vi "3d axis settings.vi"(3 "Int Current":T1, 4 "Wave Current":T1, 5 "Scan Current":T1) -> (0 "Int setting":T1, 1 "Wave setting":T1, 2 "Scan setting":T1)   [LabVIEW 2014]
panel:
  in  "Save":bool
  in  "Cancel":bool
  in  "Int Auto":bool caption="Auto"
  in  "Int Min":sgl caption="Min"
  in  "Int Max":sgl caption="Max"
  in  "Wave Auto":bool caption="Auto"
  in  "Wave Min":sgl caption="Min"
  in  "Wave Max":sgl caption="Max"
  in  "Scan Auto":bool caption="Auto"
  in  "Scan Min":sgl caption="Min"
  in  "Scan Max":sgl caption="Max"
  # "Int plot Axis scale"
  # "Wavelength"
  # "Scan"
  # "Intensity"
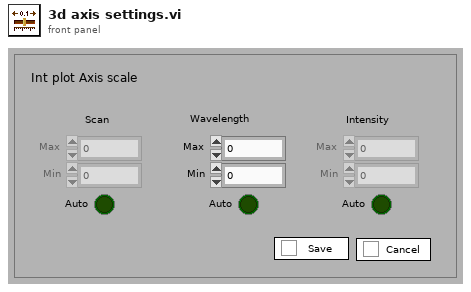
[diagram p1: front panel]
types:
  T1 = cluster{"ZScale.Maximum":dbl, "ZScale.Minimum":dbl, "ZScale.ScaleFit":u8}
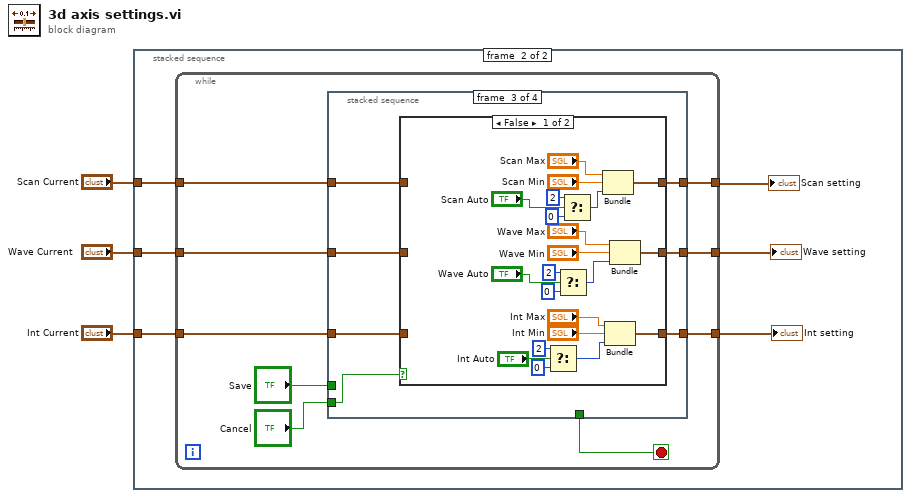
[diagram p0: block diagram]
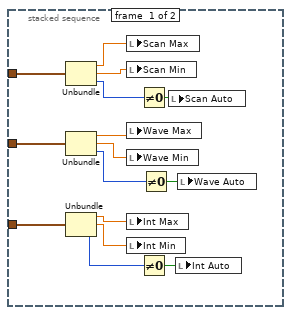
[diagram p2: hidden frame]
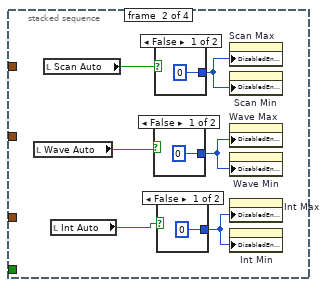
[diagram p4: hidden frame]
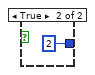
[diagram p5: hidden frame]
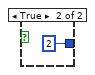
[diagram p6: hidden frame]
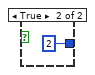
[diagram p7: hidden frame]
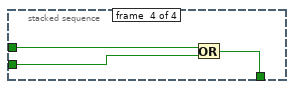
[diagram p9: hidden frame]
diagram:
  n1 = stacked-sequence {
    tunnel: "Scan Current" -> [w18 w24]
    tunnel: "Wave Current" -> [w17 w23]
    tunnel: "Int Current" -> [w16 w22]
    frame #0 {
      n2 = Unbundle(w18) -> ("ZScale.Maximum"=w15:dbl, "ZScale.Minimum"=w14:dbl, "ZScale.ScaleFit"=w9:u8)
      n3 = Unbundle(w17) -> ("ZScale.Maximum"=w13:dbl, "ZScale.Minimum"=w12:dbl, "ZScale.ScaleFit"=w7:u8)
      n4 = Unbundle(w16) -> ("ZScale.Maximum"=w11:dbl, "ZScale.Minimum"=w10:dbl, "ZScale.ScaleFit"=w5:u8)
      n5 = local write "Scan Max"(w15) -> ()
      n6 = local write "Scan Min"(w14) -> ()
      n7 = local write "Wave Max"(w13) -> ()
      n8 = local write "Wave Min"(w12) -> ()
      n9 = local write "Int Max"(w11) -> ()
      n10 = local write "Int Min"(w10) -> ()
      n11 = Not Equal To 0?(x=w9) -> (x != 0?=w8:bool)
      n12 = Not Equal To 0?(x=w5) -> (x != 0?=w4:bool)
      n13 = Not Equal To 0?(x=w7) -> (x != 0?=w6:bool)
      n14 = local write "Scan Auto"(w8) -> ()
      n15 = local write "Int Auto"(w4) -> ()
      n16 = local write "Wave Auto"(w6) -> ()
    }
    frame #1 {
      n17 = while {
        tunnel: [w33] -> w21
        tunnel: [w29] -> w20
        tunnel: [w28] -> w19
        tunnel: w24 -> [w27]
        tunnel: w23 -> [w26]
        tunnel: w22 -> [w25]
        stop <- w32 stop-if-true
        n18 = stacked-sequence {
          tunnel: [_ _ w52 _] -> w33
          tunnel: [_ _ _ w79] -> w32
          tunnel: "Cancel" -> [_ _ w49 w78]
          tunnel: "Save" -> [_ _ _ w77]
          tunnel: [_ _ w51 _] -> w29
          tunnel: [_ _ w50 _] -> w28
          tunnel: w27 -> [_ _ w48 _]
          tunnel: w26 -> [_ _ w47 _]
          tunnel: w25 -> [_ _ w46 _]
          frame #0 {
          }
          frame #1 {
            n19 = local read "Wave Auto"() -> (w37:bool)
            n20 = local read "Scan Auto"() -> (w39:bool)
            n21 = local read "Int Auto"() -> (w36:bool)
            n22 = case shown="False" w37 {
              tunnel: [0 2] -> w35
              frame False {
              }
              frame True {
              }
            }
            n23 = case shown="False" w39 {
              tunnel: [0 2] -> w38
              frame False {
              }
              frame True {
              }
            }
            n24 = case shown="False" w36 {
              tunnel: [0 2] -> w34
              frame False {
              }
              frame True {
              }
            }
            n25 = property on="Scan Max" class="DigNum (strict)"("DisabledEnum"=w38) -> ()  [unwired: 2 in, 2 out]
            n26 = property on="Scan Min" class="DigNum (strict)"("DisabledEnum"=w38) -> ()  [unwired: 2 in, 2 out]
            n27 = property on="Wave Max" class="DigNum (strict)"("DisabledEnum"=w35) -> ()  [unwired: 2 in, 2 out]
            n28 = property on="Wave Min" class="DigNum (strict)"("DisabledEnum"=w35) -> ()  [unwired: 2 in, 2 out]
            n29 = property on="Int Max" class="DigNum (strict)"("DisabledEnum"=w34) -> ()  [unwired: 2 in, 2 out]
            n30 = property on="Int Min" class="DigNum (strict)"("DisabledEnum"=w34) -> ()  [unwired: 2 in, 2 out]
          }
          frame #2 {
            n31 = case shown="False" w49 {
              tunnel: [w71 w76] -> w52
              tunnel: [w66 w75] -> w51
              tunnel: [w65 w74] -> w50
              tunnel: w48 -> [_ w76]
              tunnel: w47 -> [_ w75]
              tunnel: w46 -> [_ w74]
              frame False {
                n32 = Select(t=2, s="Int Auto", f=0) -> (s? t:f=w61:i32)
                n33 = Select(t=2, s="Wave Auto", f=0) -> (s? t:f=w53:i32)
                n34 = Select(t=2, s="Scan Auto", f=0) -> (s? t:f=w55:i32)
                n35 = Bundle("Scan Max"="Scan Max", "Scan Min"="Scan Min", w55) -> (w71:cluster{"Scan Max":sgl, "Scan Min":sgl, i32})  [unwired: 1 in]
                n36 = Bundle("Int Max"="Int Max", "Int Min"="Int Min", w61) -> (w65:cluster{"Int Max":sgl, "Int Min":sgl, i32})  [unwired: 1 in]
                n37 = Bundle("Wave Max"="Wave Max", "Wave Min"="Wave Min", w53) -> (w66:cluster{"Wave Max":sgl, "Wave Min":sgl, i32})  [unwired: 1 in]
              }
              frame True {
              }
            }
          }
          frame #3 {
            n38 = Or(x=w77, y=w78) -> (x .or. y?=w79:bool)
          }
        }
      }
      "Scan setting" <- w21
      "Wave setting" <- w20
      "Int setting" <- w19
    }
  }
